vi "adixen turbo pump controller.vi"() -> ()   [LabVIEW 2014]
panel:
  out "error out":errorcluster
  in  "Stop Button":bool
  in  "turbo on":bool
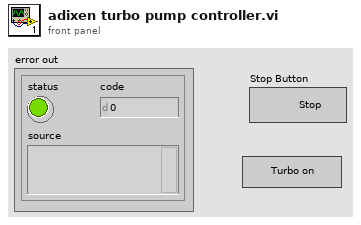
[diagram p1: front panel]
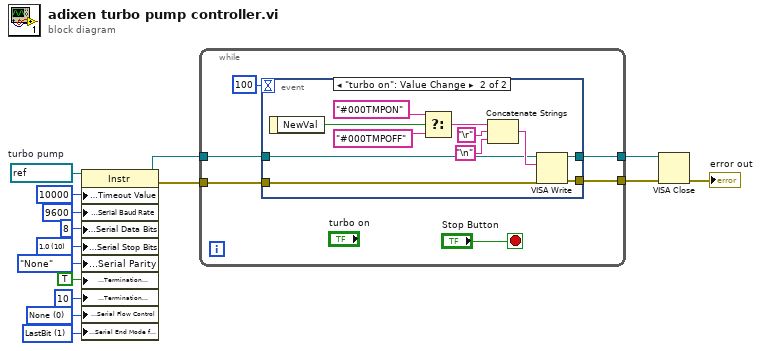
[diagram p0: block diagram]
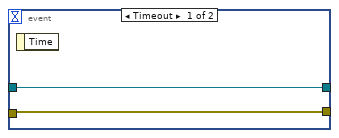
[diagram p2: hidden frame]
diagram:
  w9 = u16 1 items=["None", "LastBit", "TermChar"] ("Serial Settings:Serial End Mode for Reads")
  w7 = u16 0 items=["None", "XON/XOFF", "RTS/CTS", "XON/XOFF & RTS/CTS", "DTR/DSR", "XON/XOFF & DTR/DSR"] ("flow control (0:none)")
  w10 = u16 10 items=["1.0"=10, "1.5"=15, "2.0"=20] ("stop bits (10: 1 bit)")
  w6 = refnum<visa-resource-name> "COM7"  # turbo pump
  n1 = property class="Instr"(reference=w6, "General Settings:Timeout Value"=u32 10000 ("timeout (10sec)"), "Serial Settings:Serial Baud Rate"=u32 9600 ("baud rate (9600)"), "Serial Settings:Serial Data Bits"=u16 8 ("data bits (8)"), "Serial Settings:Serial Stop Bits"=w10, "Serial Settings:Serial Parity"=enum16{"None", "Odd", "Even", "Mark", "Space"}."None" ("parity (0:none)"), "Message Based Settings:Termination Character Enable"=TRUE ("Enable Termination\nChar (T)"), "Message Based Settings:Termination Character"=u8 10 ("termination char\n(0xA = '\\n' = LF)"), "Serial Settings:Serial Flow Control"=w7, "Serial Settings:Serial End Mode for Reads"=w9) -> (reference out=w2:refnum<visa-resource-name>, error out=w1:errorcluster)  [unwired: 1 in]
  n2 = while {
    tunnel: w1 -> [w18]
    tunnel: w2 -> [w19]
    tunnel: [w17] -> w3
    tunnel: [w16] -> w4
    stop <- "Stop Button" stop-if-true
    n3 = event shown="[1] \"turbo on\": Value Change" {
      selector: _ -> [_ _]
      dyn-events: _ -> [_ _]
      timeout: 100 -> [_ _]
      tunnel: w19 -> [w23 w27]
      tunnel: w18 -> [w22 w26]
      tunnel: [w23 w25] -> w17
      tunnel: [w22 w24] -> w16
      event Timeout {
        n4 = event-data() -> ()  [unwired: 1 in, 1 out]
      }
      event "turbo on": Value Change {
        n5 = event-data() -> ("NewVal"=w34:bool)  [unwired: 1 in]
        n6 = Select(t="#000TMPON" ("write buffer 2"), s=w34, f="#000TMPOFF" ("write buffer 2")) -> (s? t:f=w28:string)
        n7 = Concatenate Strings(w28, "\r", "\n") -> (w29:string)
        n8 = VISA Write(VISA resource name=w27, write buffer=w29, error in (no error)=w26) -> (VISA resource name out=w25:refnum<visa-resource-name>, error out=w24:errorcluster)  [unwired: 1 out]
      }
    }
  }
  n9 = VISA Close(VISA resource name=w3, error in (no error)=w4) -> (error out=→"error out":errorcluster)
